vi "Vi Tester Time Measurement.vi"() -> (2 "VI Tester report":string, 3 "VI Tester Testing time (seconds)":dbl)   [LabVIEW 2018]
uses:
  <vilib>/addons/_JKI Toolkits/VI Tester/VI Tester API.llb/Run Tests (Path).vi
  <vilib>/addons/_JKI Toolkits/VI Tester/VI Tester API.llb/VI Tester API.lvlib
panel:
  out "Project Path":string
  # "VI Tester"
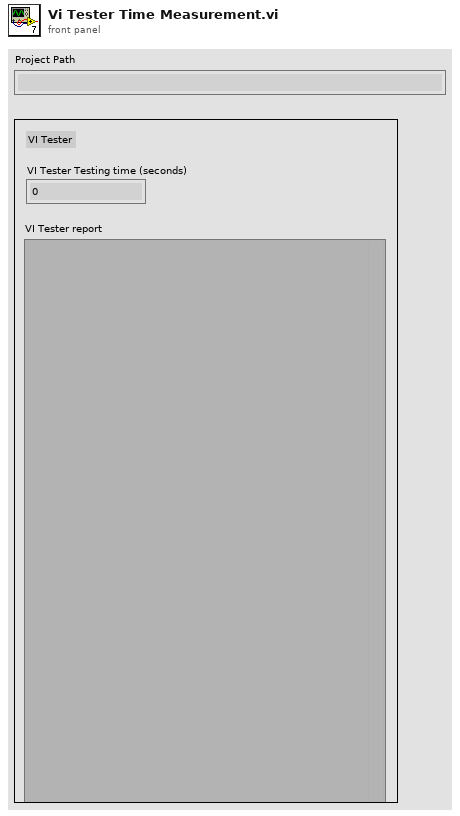
[diagram p1: front panel]
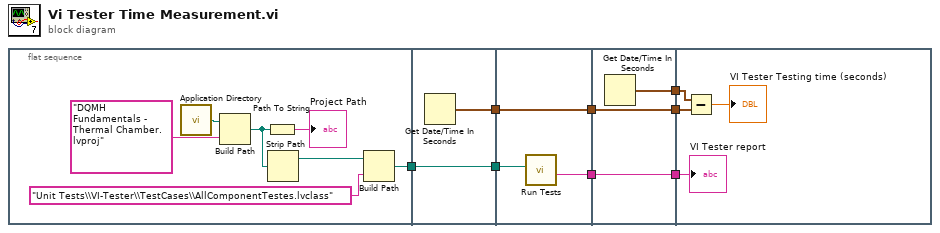
[diagram p0: block diagram]
diagram:
  n1 = flat-sequence {
    tunnel: [w10] -> w3
    tunnel: [w17] -> w8
    tunnel: [w16] -> w4
    tunnel: w3 -> [w16]
    tunnel: [w20] -> w7
    tunnel: w8 -> [w20]
    tunnel: w4 -> [w19]
    tunnel: [w18] -> w1
    tunnel: [w23] -> w6
    tunnel: [w22] -> w5
    tunnel: w7 -> [w22]
    tunnel: [w21] -> w2
    tunnel: w1 -> [w21]
    tunnel: w6 -> [w25]
    tunnel: w5 -> [w26]
    tunnel: w2 -> [w24]
    frame #0 {
      n2 = call <vilib>:"Application Directory.vi"() -> ("Application Directory"=w9:path)
      n3 = Build Path(base path=w9, name or relative path="DQMH Fundamentals - Thermal Chamber.lvproj") -> (appended path=w11:path)
      n4 = Path To String(path=w11) -> (string=→"Project Path":string)
      n5 = Strip Path(path=w11) -> (stripped path=w13:path)  [unwired: 1 out]
      n6 = Build Path(base path=w13, name or relative path="Unit Tests\\VI-Tester\\TestCases\\AllComponentTestes.lvclass") -> (appended path=w10:path)
    }
    frame #1 {
      n7 = Get Date/Time In Seconds() -> (seconds since 1Jan1904=w17:timestamp)
    }
    frame #2 {
      n8 = call-poly <vilib>:"Run Tests.vi"("Test Path"=w19) -> ("test details"=w18:string)  [unwired: 8 in, 2 out]
    }
    frame #3 {
      n9 = Get Date/Time In Seconds() -> (seconds since 1Jan1904=w23:timestamp)
    }
    frame #4 {
      n10 = Subtract(x=w25, y=w26) -> (x-y=→"VI Tester Testing time (seconds)":dbl)
      "VI Tester report" <- w24
    }
  }
